vi "TAF Parse.vi"(6 "Classes":refnum<class "Class.lvclass">[](array[class]), 11 "TargetItem in":refnum<vi>) -> (3 "TAFInterfaceConfigurations":refnum<class "TAFConfiguration.lvclass">[](array[class]))   [LabVIEW 2021, in "TAF Proj Document Type.lvlib" / "Project Parser.lvlib"]
uses:
  <vilib>/Wovalab/AntiDoc/Document Type/Add-ons/LabVIEW TAF Project/Project Parser/Project Parser.lvlib
  <vilib>/Wovalab/AntiDoc/Document Type/Add-ons/LabVIEW TAF Project/TAFConfiguration/TAFConfiguration.lvclass
  C:/Program Files (x86)/National Instruments/LabVIEW 2021/vi.lib/Wovalab/AntiDoc/Bloc/Bloc.lvclass
  <vilib>/Wovalab/AntiDoc/Document Type/Add-ons/LabVIEW TAF Project/Class/Class.lvclass
  <vilib>/Wovalab/AntiDoc/Bloc/Bloc.lvclass/Bloc.ctl
  <vilib>/Wovalab/AntiDoc/Document Type/Add-ons/LabVIEW TAF Project/TAFConfiguration/TAFConfiguration.lvclass/TAFConfiguration.ctl
  6d75f74e-b430-4036-9ad3-48fbadf5ff17.vi
  <vilib>/Wovalab/AntiDoc/Document Type/Add-ons/LabVIEW TAF Project/TAFConfiguration/Write Uml.vi
  <vilib>/Wovalab/AntiDoc/Bloc/Write Name.vi
  <vilib>/JDP Science/JSONtext/JSON text to Variant.vi
  <vilib>/JDP Science/JSONtext/LVClass Serializer/JSONtext LVClass Serializer.lvclass
  <vilib>/JDP Science/JSONtext/Config Files/Config File.lvclass
  Localdata/Projects/TriekselSoft/TriekselsoftApplicationFramework/Source/.Externals/Tools_TAF_PlantUML/ButtonBarFlow/ButtonBarFlow/ButtonBarFlow.lvlib
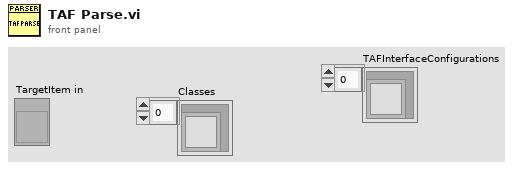
[diagram p1: front panel]
types:
  T1 = cluster{"ObjectName":string, "ObjectType":string, "Interfaces":cluster{"Label":string, "ObjectName":string, "Type":string}[]}[]
  T2 = cluster{"ObjectName":string, "ObjectFile":string, "FileContent":string}[]
  T3 = cluster{"ObjectName":string, "ObjectFile":string, "FileContent":string}
  T4 = cluster{"Captions":string[], "EnablesExpressions":string[], "ActionTypes":string[], "TargetObjects":string[], "Parameters":string[]}
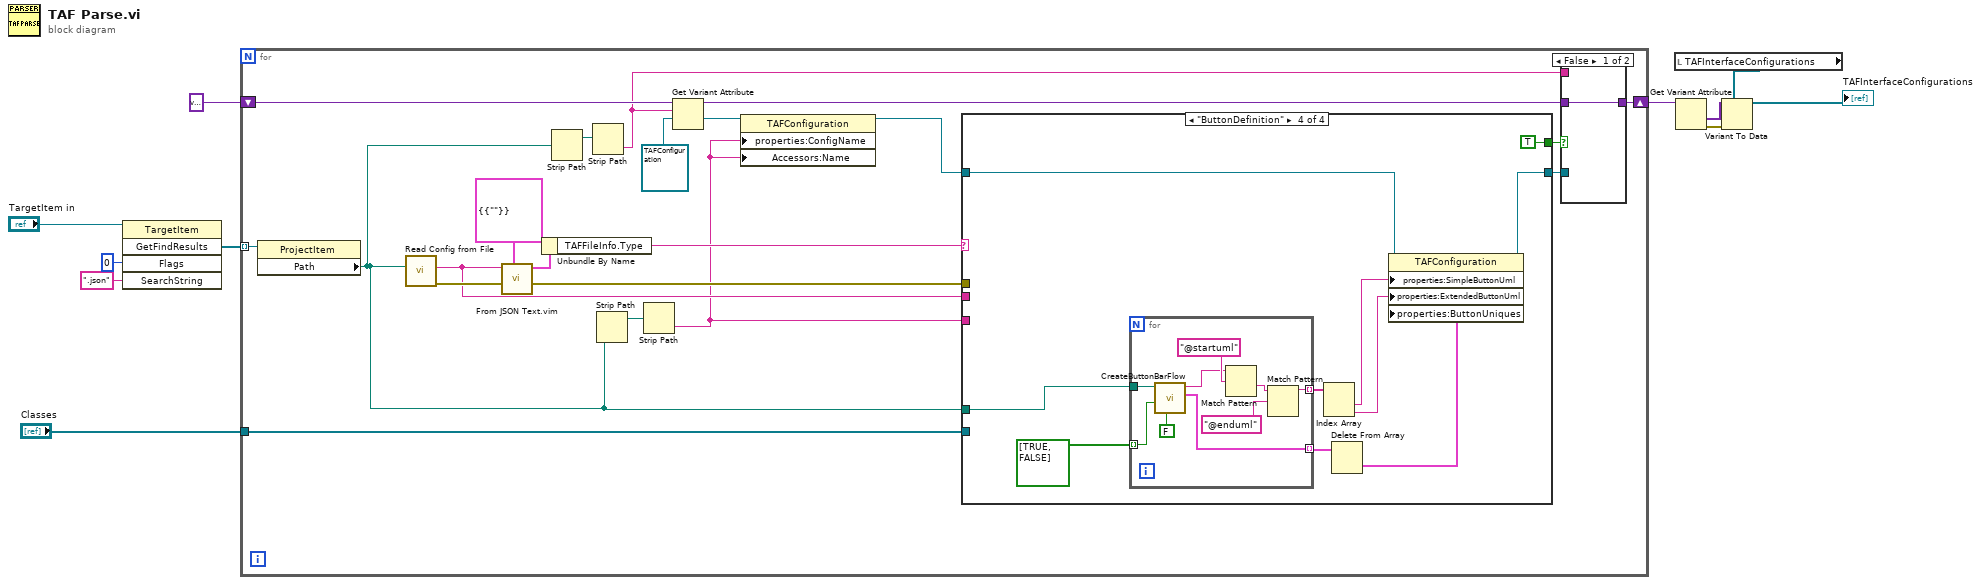
[diagram p0: block diagram]
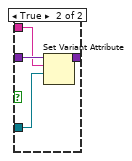
[diagram p2: hidden frame]
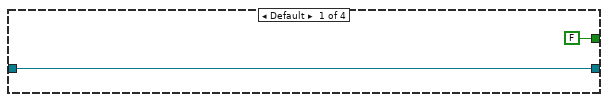
[diagram p3: hidden frame]
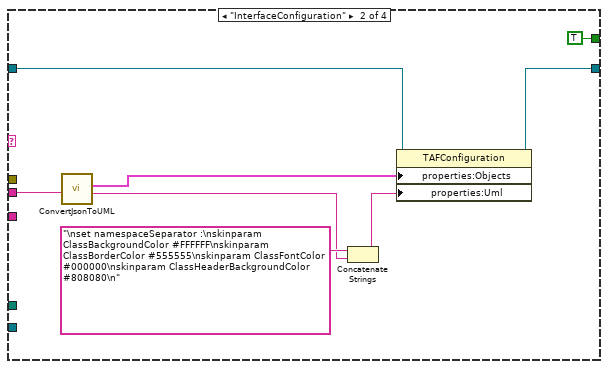
[diagram p4: hidden frame]
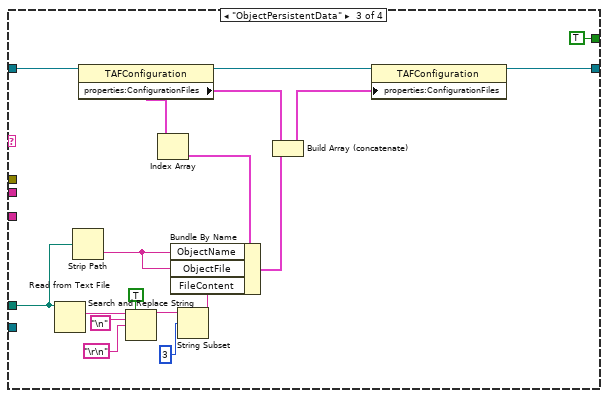
[diagram p5: hidden frame]
diagram:
  n1 = invoke class="TargetItem" method="GetFindResults"(reference="TargetItem in", "Flags"=0, "SearchString"=".json") -> ("GetFindResults"=w10:refnum<vi>[])  [unwired: 2 in, 4 out]
  n2 = for {
    tunnel: w10 -> [w32] mode=indexing
    shift-right: [w21] -> w6
    shift-left: variant -> [w25]
    tunnel: "Classes" -> [w13]
    n3 = property class="ProjectItem"(reference=w32) -> ("Path"=w15:path)  [unwired: 1 in, 2 out]
    n4 = call <vilib>:"Read Config from File.vi"("config file path"=w15) -> ("error out"=w31:errorcluster, "<JSON>Config"=w29:string)  [unwired: 7 in, 2 out]
    n5 = call "From JSON Text.vim"("Data Type and Default Value"=cluster{"TAFFileInfo":cluster{"Type":string}} {"TAFFileInfo"={"Type"=""}}, "error in (no error)"=w31, "JSON"=w29) -> ("error out"=w30:errorcluster, "Data out"=w27:cluster{"TAFFileInfo":cluster{"Type":string}})  [unwired: 7 in]
    n6 = Unbundle By Name(w27) -> ("TAFFileInfo.Type"=w17:string)
    n7 = Strip Path(path=w15) -> (stripped path=w26:path)  [unwired: 1 out]
    n8 = Strip Path(path=w26) -> (name=w20:string)  [unwired: 1 out]
    n9 = Strip Path(path=w15) -> (stripped path=w14:path)  [unwired: 1 out]
    n10 = Strip Path(path=w14) -> (name=w12:string)  [unwired: 1 out]
    n11 = Get Variant Attribute(Variant=w25, name=w20, default value (empty Variant)=refnum<class "TAFConfiguration.lvclass"> refnum ("YAFInterfaceConfiguration in")) -> (duplicate Variant=w23:variant, value=w22:refnum<class "TAFConfiguration.lvclass">)  [unwired: 1 in, 2 out]
    n12 = property class="TAFConfiguration"(reference=w22, "properties:ConfigName"=w12, "Accessors:Name"=w12) -> (reference out=w18:refnum<class "TAFConfiguration.lvclass">)  [unwired: 1 in, 1 out]
    n13 = case shown="\"ButtonDefinition\"" w17 {
      tunnel: w30 -> [_ _ _ _]
      tunnel: w29 -> [_ w47 _ _]
      tunnel: w18 -> [w39 w45 w64 w74]
      tunnel: [w39 w44 w62 w73] -> w19
      tunnel: w15 -> [_ _ w55 w68]
      tunnel: [FALSE TRUE TRUE TRUE] -> w16
      tunnel: w13 -> [_ _ _ _]
      tunnel: w12 -> [_ _ _ _]
      frame Default {
      }
      frame "InterfaceConfiguration" {
        n14 = call <vilib>:"ConvertJsonToUML.vi"("JSON"=w47) -> ("UML"=w41:string, "ObjectsS"=w46:T1)  [unwired: 9 in]
        n15 = Concatenate Strings("\nset namespaceSeparator :\nskinparam ClassBackgroundColor #FFFFFF\nskinparam ClassBorderColor #555555\nskinparam ClassFontColor #000000\nskinparam ClassHeaderBackgroundColor #808080\n" ("string"), w41) -> (w40:string)
        n16 = property class="TAFConfiguration"(reference=w45, "properties:Objects"=w46, "properties:Uml"=w40) -> (reference out=w44:refnum<class "TAFConfiguration.lvclass">)  [unwired: 1 in, 1 out]
      }
      frame "ObjectPersistentData" {
        n17 = Read from Text File(file (use dialog)=w55) -> (text=w54:string)  [unwired: 3 in, 3 out]
        n18 = Strip Path(path=w55) -> (name=w56:string)  [unwired: 1 out]
        n19 = property class="TAFConfiguration"(reference=w64) -> (reference out=w61:refnum<class "TAFConfiguration.lvclass">, "properties:ConfigurationFiles"=w59:T2)  [unwired: 1 in, 1 out]
        n20 = Search and Replace String(replace all?=TRUE ("replace all? (F)"), input string=w54, search string="\n", replace string="\r\n") -> (result string=w53:string)  [unwired: 4 in, 3 out]
        n21 = Index Array(array=w59) -> (element=w58:T3)  [unwired: 1 in]
        n22 = String Subset(string=w53, offset (0)=3) -> (substring=w49:string)  [unwired: 1 in]
        n23 = Bundle By Name(cluster=w58, "ObjectName"=w56, "ObjectFile"=w56, "FileContent"=w49) -> (w57:T3)
        n24 = Build Array (concatenate)(w59, w57) -> (w60:T2)
        n25 = property class="TAFConfiguration"(reference=w61, "properties:ConfigurationFiles"=w60) -> (reference out=w62:refnum<class "TAFConfiguration.lvclass">)  [unwired: 1 in, 1 out]
      }
      frame "ButtonDefinition" {
        n26 = for {
          tunnel: bool[] [TRUE, FALSE] -> [w77] mode=indexing
          tunnel: [w80] -> w71 mode=indexing
          tunnel: w68 -> [w79]
          tunnel: [w76] -> w66 mode=indexing
          n27 = call "CreateButtonBarFlow.vi"("ShowLegend"=FALSE, "Simplified"=w77, "Path"=w79) -> ("Uniques"=w76:T4, "PlantUMLText"=w78:string)  [unwired: 7 in]
          n28 = Match Pattern(string=w78, regular expression="@startuml") -> (after substring=w82:string)  [unwired: 1 in, 3 out]
          n29 = Match Pattern(string=w82, regular expression="@enduml") -> (before substring=w80:string)  [unwired: 1 in, 3 out]
        }
        n30 = Index Array(array=w71) -> (element #1=w70:string, element #2=w69:string)  [unwired: 2 in]
        n31 = Delete From Array(array=w66) -> (deleted portion=w65:T4)  [unwired: 2 in, 1 out]
        n32 = property class="TAFConfiguration"(reference=w74, "properties:SimpleButtonUml"=w70, "properties:ExtendedButtonUml"=w69, "properties:ButtonUniques"=w65) -> (reference out=w73:refnum<class "TAFConfiguration.lvclass">)  [unwired: 1 in, 1 out]
      }
    }
    n33 = case shown="False" w16 {
      tunnel: w23 -> [w33 w37]
      tunnel: [w33 w36] -> w21
      tunnel: w20 -> [_ w35]
      tunnel: w19 -> [_ w34]
      frame False {
      }
      frame True {
        n34 = Set Variant Attribute(Variant=w37, name=w35, value=w34) -> (Variant out=w36:variant)  [unwired: 1 in, 2 out]
      }
    }
  }
  n35 = local read "TAFInterfaceConfigurations"() -> (w3:refnum<class "TAFConfiguration.lvclass">[])
  n36 = Get Variant Attribute(Variant=w6) -> (values=w2:variant[], error out=w5:errorcluster)  [unwired: 3 in, 2 out]
  n37 = Variant To Data(error in=w5, type=w3, Variant=w2) -> (data=→"TAFInterfaceConfigurations":refnum<class "TAFConfiguration.lvclass">[])  [unwired: 1 out]
